vi "AlignTrig.vi"(10 "TRIG_REC":u32, 11 "# Samples after Trig":u16) -> (3 "Offset":u16)   [LabVIEW 2014]
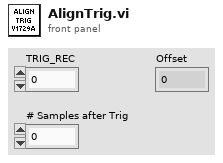
[diagram p1: front panel]
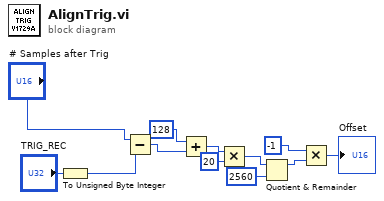
[diagram p0: block diagram]
diagram:
  n1 = To Unsigned Byte Integer(number="TRIG_REC") -> (unsigned 8bit integer=w1:u8)
  n2 = Subtract(x="# Samples after Trig", y=w1) -> (x-y=w6:u16)
  n3 = Add(x=u16 128, y=w6) -> (x+y=w8:u16)
  n4 = Multiply(x=w8, y=u16 20) -> (x*y=w10:u16)
  n5 = Quotient & Remainder(x=w10, y=u16 2560) -> (x-y*floor(x/y)=w11:u16)  [unwired: 1 out]
  n6 = Multiply(x=i16 -1, y=w11) -> (x*y=→"Offset":u16)
